vi "predict position2.vi"() -> ()   [LabVIEW 2009]
panel:
  in  "parameters":T1={"max velocity (m/s)"=2.0, "wheel base width (m)"=0.7, "traverse CoF"=0.14}
  in  "direction (rad)":dbl(knob) min=0.0 max=6.2832 step=0.03141592 scale=6.2832..0.0
  in  "resolution":i32=20
  out "output array":cluster{dbl, dbl}[](graph)
  in  "m/s":dbl(slide) scale=-2.0..2.0
  in  "time (s)":dbl(slide) scale=0.001..0.5
  # "goal of this VI:\nGraph the possible locations (relative) of the robot in the future\ngiven: time period, current speed, current turn"
  # "what the heck is it with -.3, .3, and 1.7?  This shows a very sharp turn at both of them"
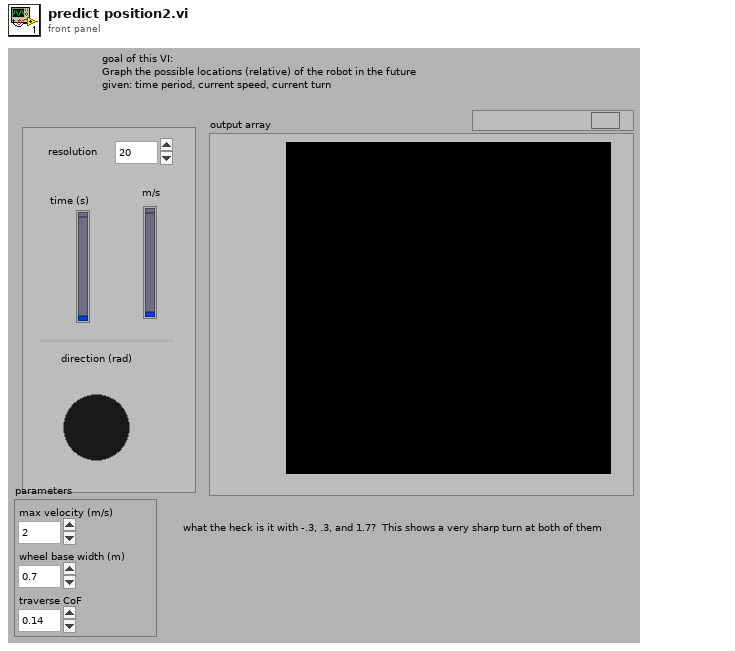
[diagram p1: front panel]
types:
  T1 = cluster{"max velocity (m/s)":dbl, "wheel base width (m)":dbl, "traverse CoF":dbl}
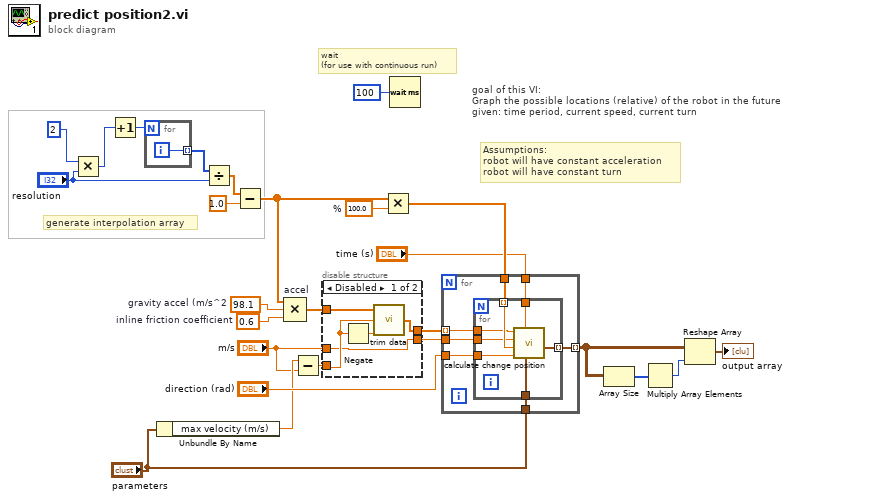
[diagram p0: block diagram]
diagram:
  w15 = 100.0  # %
  w26 = 0.6  # inline friction coefficient
  w25 = 98.1  # gravity accel (m/s^2
  # "wait\n(for use with continuous run)"
  # "Assumptions:\nrobot will have constant acceleration\nrobot will have constant turn"
  # "generate interpolation array"
  # "goal of this VI:\nGraph the possible locations (relative) of the robot in the future\ngiven: time period, current speed, current turn"
  n1 = Multiply(x=2 ("y"), y="resolution") -> (x*y=w20:i32)
  n2 = Increment(x=w20) -> (x+1=w21:i32)
  n3 = for {
    N: w21 -> [_]
    tunnel: [w27] -> w24 mode=indexing
    i -> [w27]
  }
  n4 = Unbundle By Name("parameters") -> ("max velocity (m/s)"=w3:dbl)
  n5 = Divide(x=w24, y="resolution") -> (x/y=w23:dbl[])
  n6 = Subtract(x=w23, y=1.0) -> (x-y=w16:dbl[])
  n7 = Compound Arithmetic op=MULTIPLY "accel"(w16, w25, w26) -> (w7:dbl[])
  n8 = Subtract(x=w3, y="m/s") -> (x-y=w4:dbl)
  n9 = disable-structure shown="Disabled" {
    disable-tunnel: w7 -> [w32 w34]
    disable-tunnel: [w29 w34] -> w6
    disable-tunnel: w4 -> [w30 _]
    disable-tunnel: [w28 w33] -> w2
    disable-tunnel: "m/s" -> [w28 w33]
    frame #0 {
      n10 = Negate(x=w30) -> (-x=w31:dbl)
      n11 = call "trim data.vi"("min value"=w31, "max value"=w30, "Array in"=w32) -> ("Array out"=w29:dbl[])  [unwired: 2 in]
    }
    frame #1 {
    }
  }
  n12 = Multiply(x=w16, y=w15) -> (x*y=w14:dbl[])
  n13 = Wait (ms)(milliseconds to wait=u32 100) -> ()  [unwired: 1 out]
  n14 = for {
    tunnel: w14 -> [w41]
    tunnel: "parameters" -> [w40]
    tunnel: "time (s)" -> [w39]
    tunnel: w2 -> [w38]
    tunnel: w6 -> [w37] mode=indexing
    tunnel: [w36] -> w11 mode=indexing
    tunnel: "direction (rad)" -> [w35]
    n15 = for {
      tunnel: w41 -> [w48] mode=indexing
      tunnel: w40 -> [w47]
      tunnel: w39 -> [w46]
      tunnel: w38 -> [w45]
      tunnel: w37 -> [w44]
      tunnel: [w43] -> w36 mode=indexing
      tunnel: w35 -> [w42]
      n16 = call "calculate change position.vi"("parameters"=w47, "Ætime (s)"=w46, "initial direction"=w42, "% turn"=w48, "m/s"=w45, "m/s/s"=w44) -> ("Æ point"=w43:cluster{dbl, dbl})  [unwired: 4 in, 1 out]
    }
  }
  n17 = Array Size(array=w11) -> (size(s)=w12:i32[])
  n18 = Multiply Array Elements(1:w12) -> (0:w10:i32)
  n19 = Reshape Array(w11, w10) -> (→"output array":cluster{dbl, dbl}[])
